vi "NI Programmable Power Supply Hardware Selection.vi"(3 "error in (no error)":errorcluster) -> (0 "error out":errorcluster, 1 "Power Supply NI-MAX Device Name Out":string, 2 "Power Supply In Use Out":enum16{"PXIe-4112", "PXI-4110"}(ring))   [LabVIEW 2018]
panel:
  in  "OK Button":bool
  in  "Power Supply NI-MAX Device Name":string
  in  "Power Supply In Use":enum16{"PXIe-4112", "PXI-4110"}(ring)
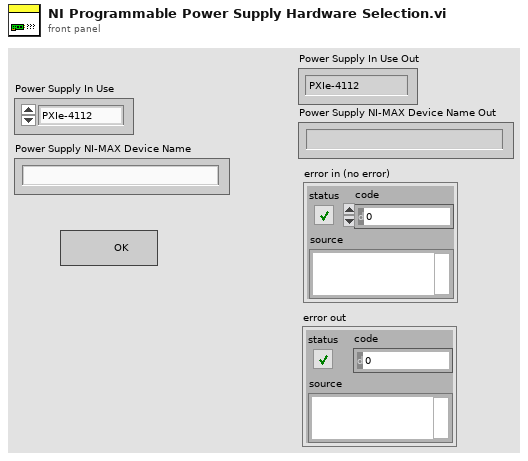
[diagram p1: front panel]
types:
  T1 = enum32{"Invalid", "Standard", "Closed", "Hidden", "Minimized", "Maximized"}
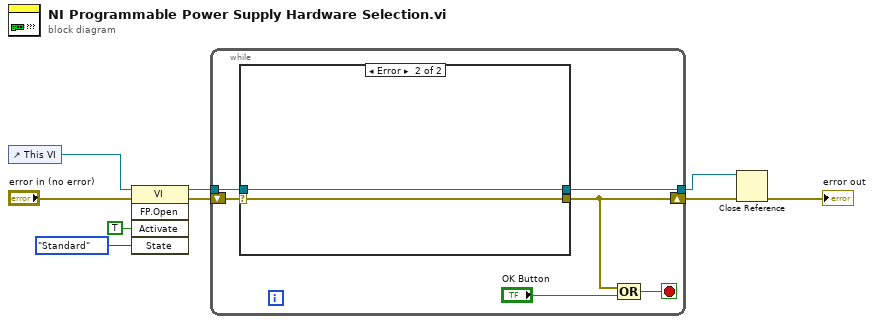
[diagram p0: block diagram]
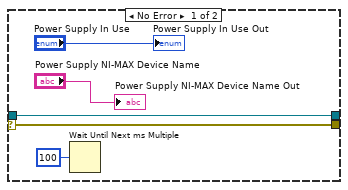
[diagram p2: hidden frame]
diagram:
  n1 = control-ref of="This VI"() -> (w9:refnum<vi>)
  n2 = invoke class="VI" method="FP.Open"(reference=w9, error in="error in (no error)", "Activate"=TRUE ("Activate?"), "State"=T1."Standard") -> (reference out=w4:refnum<vi>, error out=w6:errorcluster)  [unwired: 1 in, 3 out]
  n3 = while {
    shift-right: [w12] -> w3
    shift-left: w6 -> [w15]
    tunnel: w4 -> [w11]
    tunnel: [w10] -> w2
    stop <- w13 stop-if-true
    n4 = case shown="Error" w15 {
      selector: w15 -> [w17 w22]
      tunnel: [w17 w22] -> w12
      tunnel: w11 -> [w16 w21]
      tunnel: [w16 w21] -> w10
      frame No Error {
        n5 = Wait Until Next ms Multiple(millisecond multiple=u32 100) -> ()  [unwired: 1 out]
        "Power Supply In Use Out" <- "Power Supply In Use"
        "Power Supply NI-MAX Device Name Out" <- "Power Supply NI-MAX Device Name"
      }
      frame Error {
      }
    }
    n6 = Compound Arithmetic op=OR(w12, "OK Button") -> (w13:bool)
  }
  n7 = Close Reference(reference=w2, error in (no error)=w3) -> (error out=→"error out":errorcluster)
